vi "Start DO.vi"(0 "reference in":refnum<class "DO.lvclass">, 5 "error in (no error)":errorcluster) -> (14 "reference out":refnum<class "DO.lvclass">, 19 "error out":errorcluster)   [LabVIEW 2017, in "DO.lvclass"]
uses:
  DO.lvclass
  utils/DO_Write.vi
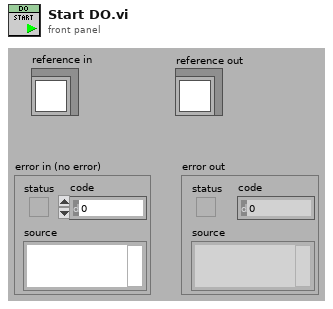
[diagram p1: front panel]
types:
  T1 = typedef "DO.lvclass/ObjectAttributes.ctl" = cluster{"DO Task":refnum<k21>, "DO Module Names (NI-Max Name)":string[], "Number of Channels Per DO Module":i32[], "DO Status":bool[], "Number of DO Modules":u32, "DO Status to Set":bool[], "DO On/Off Status":bool, "DO VI Reference":refnum<vi>, "Number of Total DO Channels":u32}
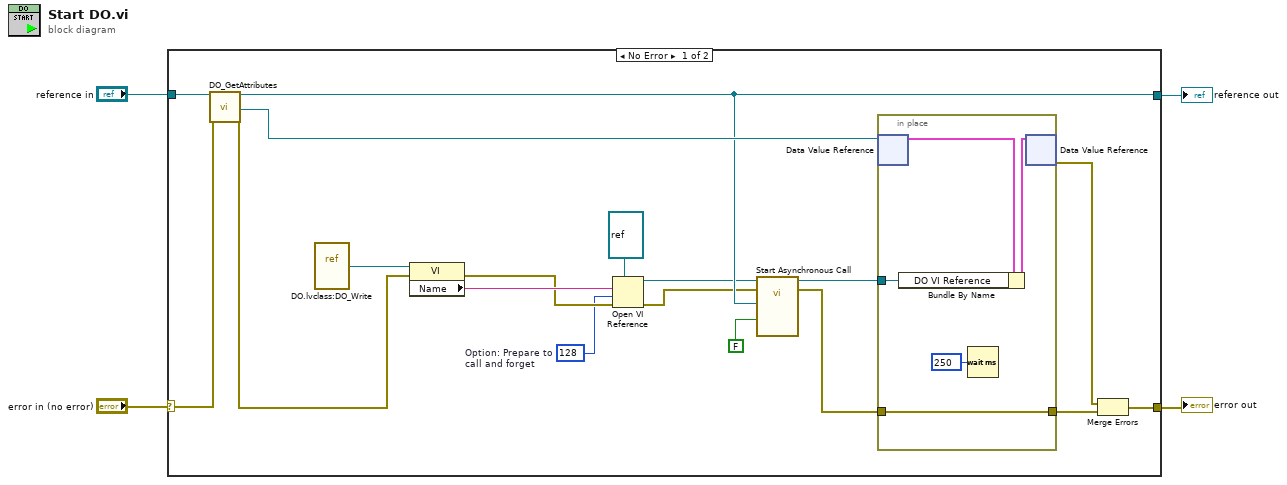
[diagram p0: block diagram]
diagram:
  n1 = case shown="No Error" "error in (no error)" {
    selector: "error in (no error)" -> [w21 w29]
    tunnel: [w19 w29] -> w3
    tunnel: [w11 w28] -> w1
    tunnel: "reference in" -> [w22 w28]
    frame No Error {
      w9 = 128  # Option: Prepare to  call and forget
      n2 = call "DO_GetAttributes.vi"("reference in"=w22, "error in (no error)"=w21) -> ("reference out"=w11:refnum<class "DO.lvclass">, "DataRef"=w18:refnum<data-value>, "error out"=w10:errorcluster)  [unwired: 14 in, 1 out]
      n3 = vi-ref "DO.lvclass:DO_Write.vi"() -> (w14:refnum<vi>)
      n4 = property class="VI"(reference=w14, error in=w10) -> (error out=w13:errorcluster, "Name"=w15:string)  [unwired: 1 out]
      n5 = Open VI Reference(type specifier VI Refnum (for type only)=refnum<vi> refnum, vi path=w15, options=w9, error in (no error)=w13) -> (vi reference=w6:refnum<vi>, error out=w5:errorcluster)  [unwired: 2 in]
      n6 = call-by-ref "Start Asynchronous Call"(reference=w6, error in=w5, "reference in"=w11, "Stop DO"=FALSE ("Stop Timer")) -> (reference out=w8:refnum<vi>, error out=w7:errorcluster)  [unwired: 7 in, 2 out]
      n7 = in-place {
        in-place-border: w7 -> [w25]
        in-place-border: [w25] -> w17
        in-place-border: w8 -> [w24]
        n8 = in-place-dvr #1(w18) -> (w26:T1)  [unwired: 1 out]
        n9 = Bundle By Name(cluster=w26, "DO VI Reference"=w24) -> (w27:T1)
        n10 = Wait (ms)(milliseconds to wait=u32 250) -> ()  [unwired: 1 out]
        n11 = in-place-dvr #1(w27) -> (w20:errorcluster)  [unwired: 1 out]
      }
      n12 = Merge Errors(w20, w17) -> (w19:errorcluster)
    }
    frame Error {
    }
  }
  "error out" <- w3
  "reference out" <- w1
